vi "军蚁-保存历史图片铜环.vi"(7 "类型":string(combo), 8 "error in (no error)":errorcluster, 9 "Image in":T1(plugin-control), 10 "NGOK":string(combo), 11 "基路径":path) -> (0 "error out":errorcluster)   [LabVIEW 2017]
panel:
  out "连接的字符串 2":string
  out "连接的字符串":string
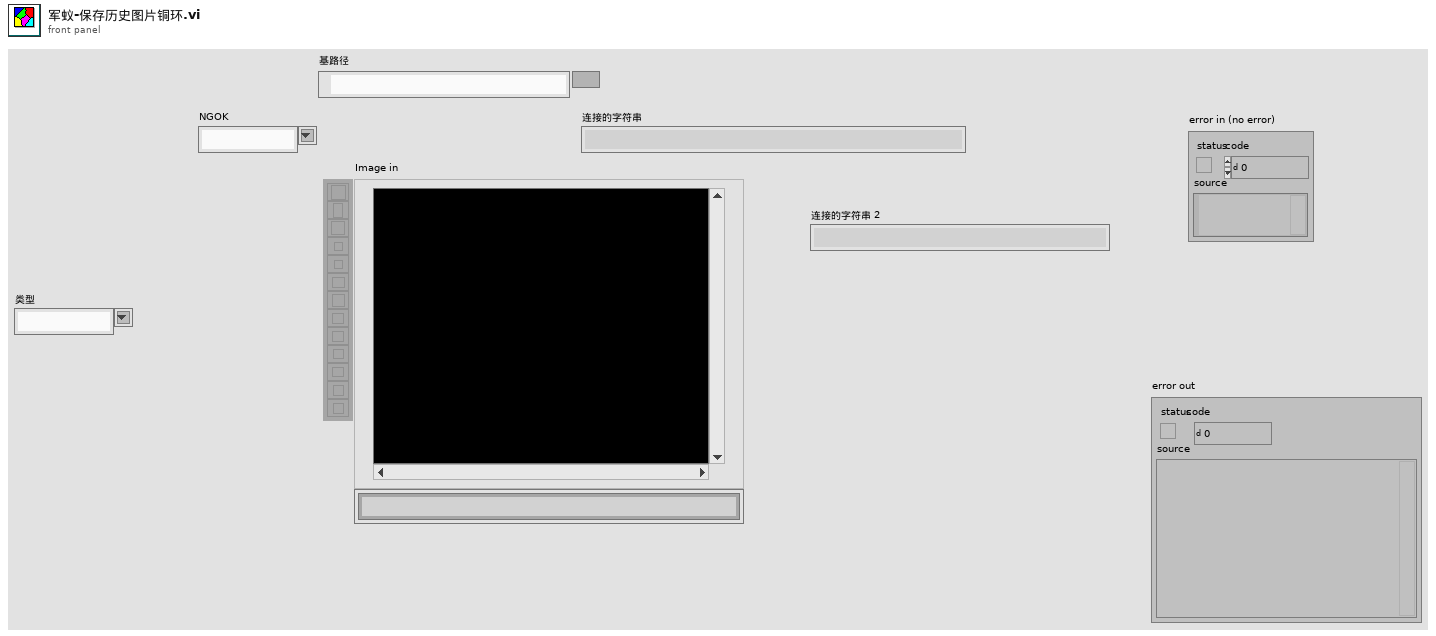
[diagram p1: front panel]
types:
  T1 = typedef "IMAQ Image.ctl" = refnum<image>
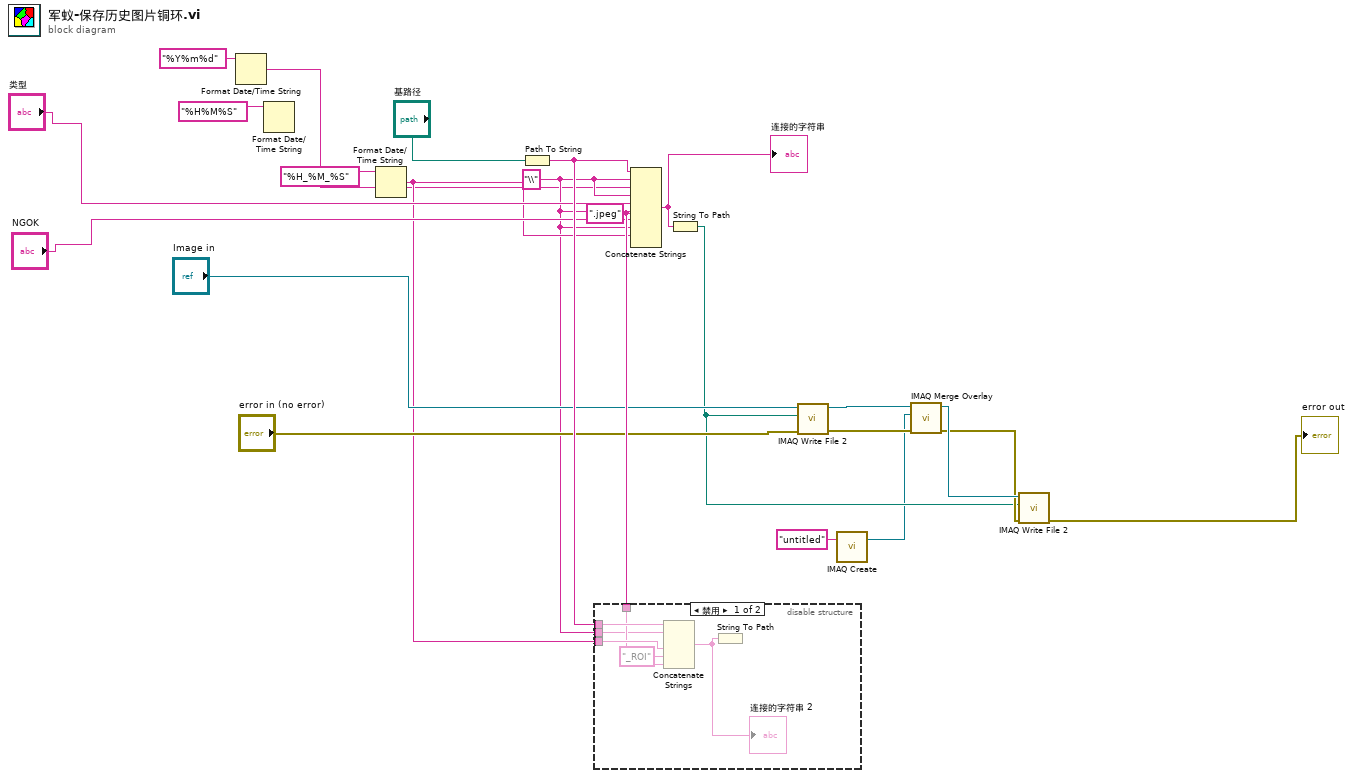
[diagram p0: block diagram]
diagram:
  w18 = ".jpeg" ("字符串")
  w7 = "\\" ("字符串")
  n1 = Format Date/Time String(time format string (%c)="%Y%m%d" ("时间格式字符串(%c)")) -> (date/time string=w5:string)  [unwired: 2 in]
  n2 = Format Date/Time String(time format string (%c)="%H%M%S" ("时间格式字符串(%c)")) -> ()  [unwired: 2 in, 1 out]
  n3 = Format Date/Time String(time format string (%c)="%H_%M_%S" ("时间格式字符串(%c)")) -> (date/time string=w8:string)  [unwired: 2 in]
  n4 = Path To String(path="基路径") -> (string=w19:string)
  n5 = disable-structure shown="禁用" {
    disable-tunnel: w19 -> [w28 _]
    disable-tunnel: w8 -> [w27 _]
    disable-tunnel: w18 -> [w26 _]
    disable-tunnel: w7 -> [w25 _]
    frame Disabled {
      n6 = Concatenate Strings(w28, w25, w27, "_ROI" ("字符串"), w26) -> (w23:string)  [unwired: 1 in]
      "连接的字符串 2" <- w23
      n7 = String To Path(string=w23) -> ()  [unwired: 1 out]
    }
    frame Enabled {
    }
  }
  n8 = Concatenate Strings(w19, w7, w5, w7, "类型", w7, "NGOK", w7, w8, w18) -> (w20:string)
  "连接的字符串" <- w20
  n9 = String To Path(string=w20) -> (path=w10:path)
  n10 = call-poly "IMAQ Write File 2"("error in (no error)"="error in (no error)", "File Path"=w10, "Image"="Image in") -> ("error out"=w3:errorcluster, "Image Out (duplicate)"=w4:T1)  [unwired: 7 in]
  n11 = call "IMAQ Create"("Image Name"="untitled") -> ("New Image"=w1:T1)  [unwired: 4 in, 1 out]
  n12 = call "IMAQ Merge Overlay"("error in (no error)"=w3, "Image Dst"=w1, "Image Src"=w4) -> ("error out"=w12:errorcluster, "Image Dst Out"=w14:T1)  [unwired: 7 in]
  n13 = call-poly "IMAQ Write File 2"("error in (no error)"=w12, "File Path"=w10, "Image"=w14) -> ("error out"=→"error out":errorcluster)  [unwired: 7 in, 1 out]
